vi "Build_Web_Services.vi"(8 "error in (no error)":errorcluster, 11 "Installer in":refnum<class "Installer.lvclass">) -> (0 "error out":errorcluster, 3 "Installer out":refnum<class "Installer.lvclass">)   [LabVIEW 2020, in "Installer.lvclass"]
uses:
  <vilib>/AppBuilder/IB_Classes/Installer/Installer.lvclass
  <vilib>/AppBuilder/IB_Classes/Installer/Installer.lvclass/Installer.ctl
  <vilib>/AppBuilder/IB_Classes/Destination/IB_Destination.lvclass
  <vilib>/AppBuilder/IB_Classes/Source/IB_Source.lvclass
  <resource>/Framework/Providers/Builds/Installer/CDK_GLOBAL_LABELS.vi
  <vilib>/AppBuilder/IB_Classes/Source/File_Web_Service/IB_Source_File_Web_Service.lvclass
  C:/Program Files (x86)/National Instruments/LabVIEW 2020/vi.lib/AppBuilder/IB_Classes/Source/File/IB_Source_File.lvclass
  C:/Program Files (x86)/National Instruments/LabVIEW 2020/vi.lib/AppBuilder/IB_Classes/Source/IB_Source.lvclass
  C:/Program Files (x86)/National Instruments/LabVIEW 2020/vi.lib/AppBuilder/IB_Classes/Source/File_Web_Service/IB_Source_File_Web_Service.lvclass
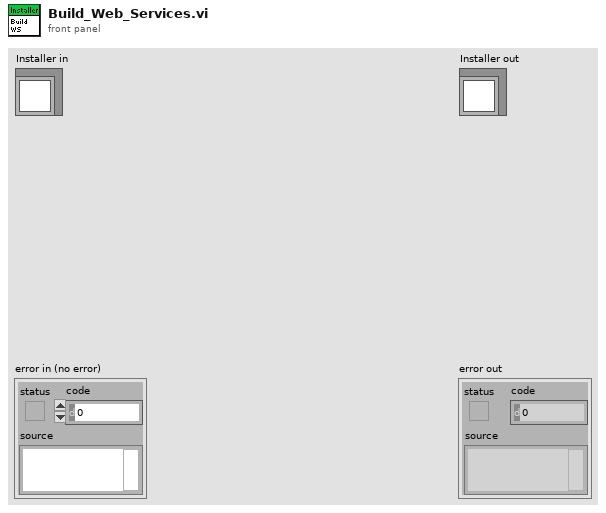
[diagram p1: front panel]
types:
  T1 = enum32{"NI Web Server", "Application Web Server"}
  T2 = typedef "ItemRef.ctl" = u64
  T3 = typedef "IB_Destination.ctl" = cluster{"name":string, "unlock":bool, "parentTag":string, "destTag":string, "eng_installPath":string}
  T4 = typedef "IB_Source.ctl" = cluster{"name":string, "sourceTag":string, "destTag":string, "path":path, "eng_installPath":string, "UI_inBuild?":bool, "str ref?":bool}
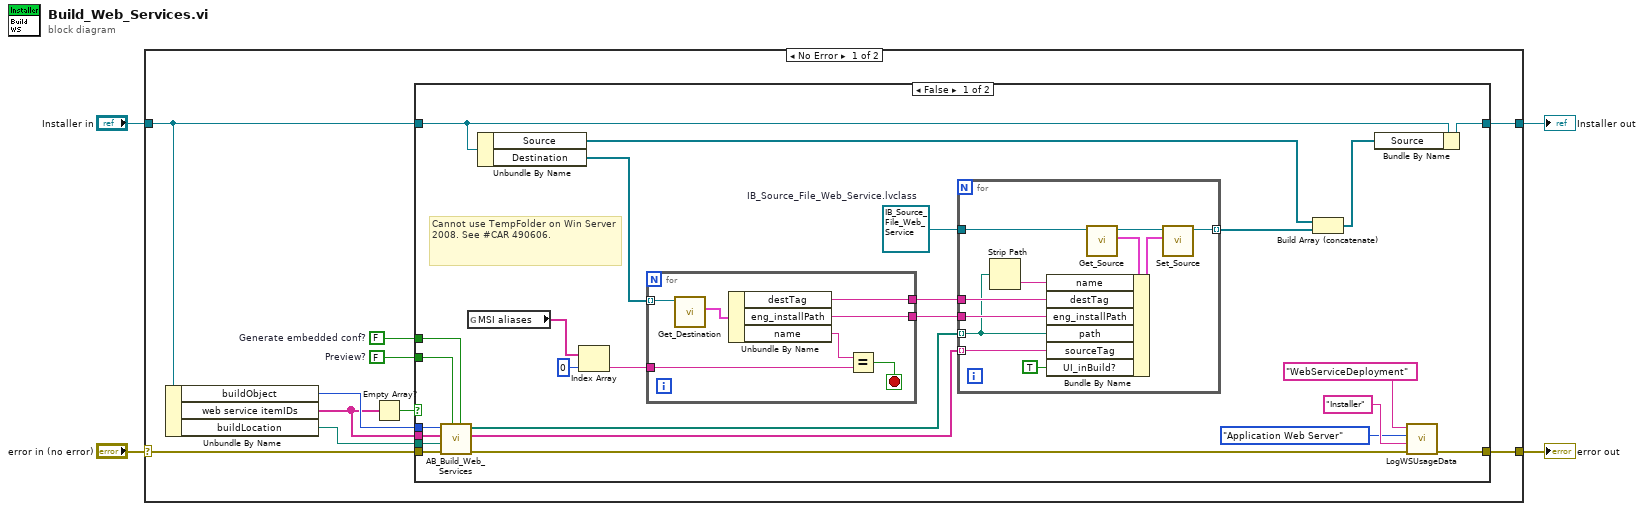
[diagram p0: block diagram]
diagram:
  n1 = case shown="No Error" "error in (no error)" {
    selector: "error in (no error)" -> [w14 w61]
    tunnel: [w13 w61] -> w3
    tunnel: [w7 w60] -> w1
    tunnel: "Installer in" -> [w8 w60]
    frame No Error {
      w6 = FALSE  # Generate embedded conf?
      w5 = FALSE  # Preview?
      n2 = Unbundle By Name(w8) -> ("buildObject"=w12:T2, "web service itemIDs"=w9:string[], "buildLocation"=w11:path)
      n3 = Empty Array?(array=w9) -> (empty?=w10:bool)
      n4 = case shown="False" w10 {
        tunnel: w14 -> [w39 w59]
        tunnel: [w16 w59] -> w13
        tunnel: w12 -> [w38 _]
        tunnel: w9 -> [w37 _]
        tunnel: w11 -> [w36 _]
        tunnel: [w32 w58] -> w7
        tunnel: w8 -> [w33 w58]
        tunnel: w6 -> [w35 _]
        tunnel: w5 -> [w34 _]
        frame False {
          w20 = refnum<class "IB_Source_File_Web_Service.lvclass"> refnum  # IB_Source_File_Web_Service.lvclass
          # "Cannot use TempFolder on Win Server 2008. See #CAR 490606."
          n5 = call <vilib>:"AB_Build_Web_Services.vi"("Generate embedded conf?"=w35, "Preview?"=w34, "error in (no error)"=w39, "Destination directory"=w36, "web service itemIDs"=w37, "build object"=w38) -> ("error out"=w17:errorcluster, "GeneratedFileGUIDs"=w25:string[], "GeneratedFiles"=w28:path[])  [unwired: 3 in]
          n6 = global read "CDK_GLOBAL_LABELS.vi" "MSI aliases"() -> (w23:string[])
          n7 = Unbundle By Name(w33) -> ("Source"=w30:refnum<class "IB_Source.lvclass">[], "Destination"=w31:refnum<class "IB_Destination.lvclass">[])
          n8 = Index Array(array=w23, index=0) -> (element=w21:string)
          n9 = for {
            tunnel: w31 -> [w57] mode=indexing
            tunnel: w21 -> [w55]
            tunnel: [w53] -> w27
            tunnel: [w52] -> w26
            stop <- w54 stop-if-true
            n10 = call <vilib>:"Get_Destination.vi"("IB_Destination in"=w57) -> ("data"=w56:T3)  [unwired: 8 in, 2 out]
            n11 = Unbundle By Name(w56) -> ("destTag"=w52:string, "eng_installPath"=w53:string, "name"=w51:string)
            n12 = Equal?(x=w51, y=w55) -> (x = y?=w54:bool)
          }
          n13 = for {
            tunnel: w28 -> [w44] mode=indexing
            tunnel: w27 -> [w46]
            tunnel: w26 -> [w47]
            tunnel: w25 -> [w45] mode=indexing
            tunnel: [w41] -> w24 mode=indexing
            tunnel: w20 -> [w40]
            n14 = Strip Path(path=w44) -> (name=w43:string)  [unwired: 1 out]
            n15 = call <vilib>:"Get_Source.vi"("IB_Source in"=w40) -> ("data"=w49:T4, "IB_Source out"=w50:refnum<class "IB_Source_File_Web_Service.lvclass">)  [unwired: 8 in, 1 out]
            n16 = Bundle By Name(cluster=w49, "name"=w43, "destTag"=w47, "eng_installPath"=w46, "path"=w44, "sourceTag"=w45, "UI_inBuild?"=TRUE) -> (w48:T4)
            n17 = call <vilib>:"Set_Source.vi"("data"=w48, "IB_Source in"=w50) -> ("IB_Source out"=w41:refnum<class "IB_Source_File_Web_Service.lvclass">)  [unwired: 8 in, 1 out]
          }
          n18 = Build Array (concatenate)(w30, w24) -> (w29:refnum<class "IB_Source.lvclass">[])
          n19 = Bundle By Name(cluster=w33, "Source"=w29) -> (w32:refnum<class "Installer.lvclass">)
          n20 = call <vilib>:"LogWSUsageData.vi"("Error In"=w17, "Deploy Method"="Installer", "Server Type"=T1."Application Web Server", "Action"="WebServiceDeployment") -> ("Error Out"=w16:errorcluster)  [unwired: 7 in]
        }
        frame True {
        }
      }
    }
    frame Error {
    }
  }
  "error out" <- w3
  "Installer out" <- w1
